vi "FTW-JSON-MergeStrings.vi"(8 "error in (no error)":errorcluster, 9 "Initial JSON String (\"\")":string, 10 "JSON string to merge (\"\")":string, 11 "Update Mode (0: Upsert)":T1) -> (0 "error out":errorcluster, 3 "Merged JSON String (UTF-8)":string)   [LabVIEW 2015]
doc: "This VI merges two JSON strings together."
uses:
  FTW-JSON-UpdateMode.ctl
  FTW-JSON.lvclass
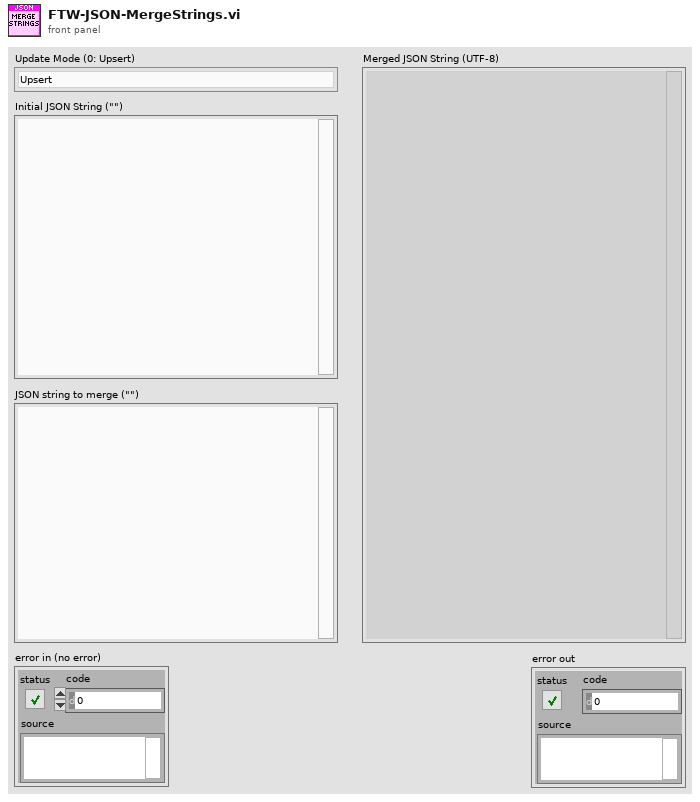
[diagram p1: front panel]
types:
  T1 = typedef "FTW-JSON.lvclass/FTW-JSON-UpdateMode.ctl" = enum16{"Upsert", "Update Only", "Insert Only"}
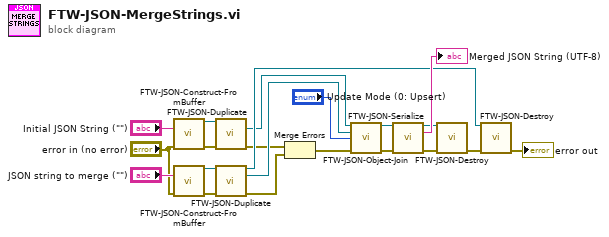
[diagram p0: block diagram]
diagram:
  n1 = call "FTW-JSON-Construct-FromBuffer.vi"("JSON String (UTF-8)"="Initial JSON String (\"\")", "error in"="error in (no error)") -> ("JSON Object"=w7:refnum<class "FTW-JSON.lvclass">, "error out"=w5:errorcluster)  [unwired: 12 in]
  n2 = call "FTW-JSON-Construct-FromBuffer.vi"("JSON String (UTF-8)"="JSON string to merge (\"\")", "error in"="error in (no error)") -> ("JSON Object"=w10:refnum<class "FTW-JSON.lvclass">, "error out"=w3:errorcluster)  [unwired: 12 in]
  n3 = call "FTW-JSON-Duplicate.vi"("JSON Object"=w7, "error in"=w5) -> ("Duplicated JSON Object"=w6:refnum<class "FTW-JSON.lvclass">, "error out"=w4:errorcluster)  [unwired: 11 in, 1 out]
  n4 = call "FTW-JSON-Duplicate.vi"("JSON Object"=w10, "error in"=w3) -> ("JSON Object out"=w9:refnum<class "FTW-JSON.lvclass">, "Duplicated JSON Object"=w8:refnum<class "FTW-JSON.lvclass">, "error out"=w2:errorcluster)  [unwired: 11 in]
  n5 = Merge Errors(w4, w2) -> (w16:errorcluster)
  n6 = call "FTW-JSON-Object-Join.vi"("JSON Object"=w6, "JSON Object to Merge"=w8, "Join Mode"="Update Mode (0: Upsert)", "error in"=w16) -> ("JSON Object out"=w13:refnum<class "FTW-JSON.lvclass">, "error out"=w14:errorcluster)  [unwired: 10 in]
  n7 = call "FTW-JSON-Serialize.vi"("JSON Object"=w13, "error in"=w14) -> ("JSON Object out"=w19:refnum<class "FTW-JSON.lvclass">, "JSON String (UTF-8)"=→"Merged JSON String (UTF-8)":string, "error out"=w18:errorcluster)  [unwired: 11 in]
  n8 = call "FTW-JSON-Destroy.vi"("JSON Object"=w19, "error in"=w18) -> ("error out"=w12:errorcluster)  [unwired: 13 in]
  n9 = call "FTW-JSON-Destroy.vi"("JSON Object"=w9, "error in"=w12) -> ("error out"=→"error out":errorcluster)  [unwired: 13 in]
